vi "RTM - Add Packet.vi"() -> ()   [LabVIEW 2015, in "UDP-Custom-Device System Explorer.lvlib"]
uses:
  UDP-Custom-Device System Explorer.lvlib
  Shared/Constants.vi
  <vilib>/NI Veristand/Custom Device API/Get Item Property (String Array).vi
  <vilib>/NI Veristand/Custom Device API/Set Item Property (String Array).vi
  <vilib>/NI VeriStand/Custom Device API/Custom Device API.lvlib
  Shared/UDP-Custom-Device Shared.lvlib
  <vilib>/NI VeriStand/Custom Device Tools/Custom Device Utility Library/Custom Device Utility Library.lvlib
panel:
  in  "Cancel Button":bool
  in  "OK Button":bool
  in  "New Packet ID":string
  in  "New Packet Name":string
  in  "Tag":string
  in  "Node Ptr":u64 format="%.0x"
  out "error out":errorcluster
  in  "error in (no error)":errorcluster
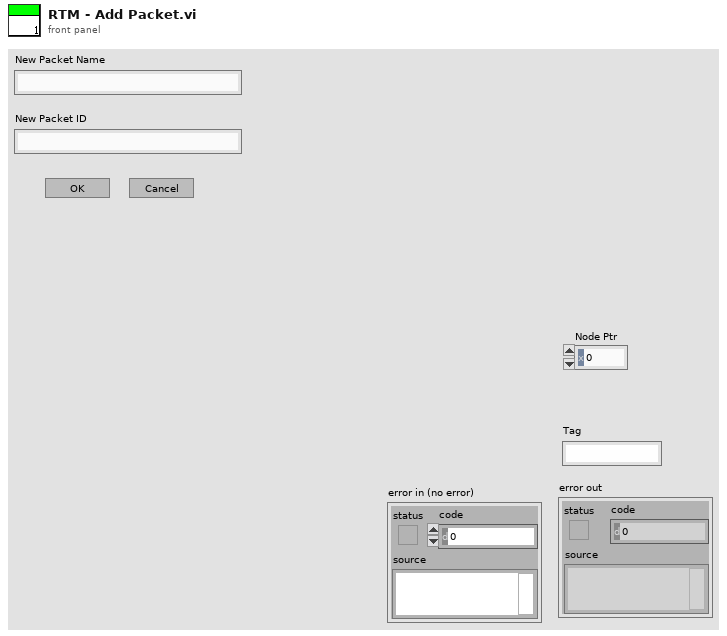
[diagram p1: front panel]
types:
  T1 = enum32{"Invalid", "Standard", "Closed", "Hidden", "Minimized", "Maximized"}
  T2 = typedef "Custom Device API.lvlib/Custom Device Item Ref.ctl" = u64
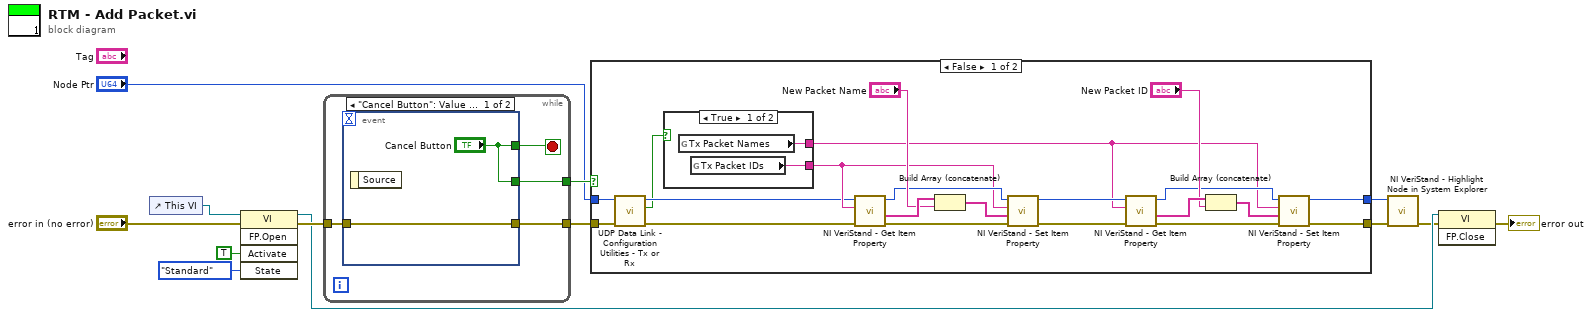
[diagram p0: block diagram]
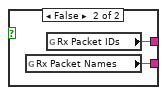
[diagram p2: hidden frame]
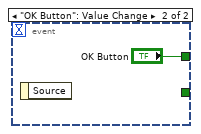
[diagram p4: hidden frame]
diagram:
  n1 = control-ref of="This VI"() -> (w13:refnum<vi>)
  n2 = invoke class="VI" method="FP.Open"(reference=w13, error in="error in (no error)", "Activate"=TRUE ("Activate?"), "State"=T1."Standard") -> (reference out=w4:refnum<vi>, error out=w9:errorcluster)  [unwired: 1 in, 3 out]
  n3 = while {
    tunnel: w9 -> [w16]
    tunnel: [w15] -> w7
    tunnel: [w14] -> w8
    stop <- w17 stop-if-true
    n4 = event shown="[0] \"Cancel Button\": Value Change" {
      selector: _ -> [_ _]
      dyn-events: _ -> [_ _]
      timeout: _ -> [_ _]
      tunnel: ["Cancel Button" "OK Button"] -> w17
      tunnel: w16 -> [w19 _]
      tunnel: [w19 _] -> w15
      tunnel: ["Cancel Button" _] -> w14
      event "Cancel Button": Value Change {
        n5 = event-data() -> ()  [unwired: 1 in, 1 out]
      }
      event "OK Button": Value Change {
        n6 = event-data() -> ()  [unwired: 1 in, 1 out]
      }
    }
  }
  n7 = case shown="False" w8 {
    tunnel: w7 -> [w25 w47]
    tunnel: [w31 w47] -> w3
    tunnel: "Node Ptr" -> [w26 w46]
    tunnel: [w21 w46] -> w1
    frame False {
      n8 = call "UDP Data Link - Configuration Utilities - Tx or Rx.vi"("error in (no error)"=w25, "Item Ref in"=w26) -> ("error out"=w24:errorcluster, "Tx?"=w22:bool, "Item Ref out"=w23:T2)  [unwired: 7 in]
      n9 = case shown="True" w22 {
        tunnel: [w43 w45] -> w28
        tunnel: [w42 w44] -> w27
        frame True {
          n10 = global read "Constants.vi" "Tx Packet Names"() -> (w42:string)
          n11 = global read "Constants.vi" "Tx Packet IDs"() -> (w43:string)
        }
        frame False {
          n12 = global read "Constants.vi" "Rx Packet Names"() -> (w45:string)
          n13 = global read "Constants.vi" "Rx Packet IDs"() -> (w44:string)
        }
      }
      n14 = call-poly <vilib>:"NI VeriStand - Get Item Property.vi"("error in (no error)"=w24, "Property Name"=w28, "Item Ref in"=w23) -> ("error out"=w41:errorcluster, "Value"=w40:string[], "Item Ref out"=w30:T2)  [unwired: 5 in, 1 out]
      n15 = Build Array (concatenate)(w40, "New Packet Name") -> (w39:string[])
      n16 = call-poly <vilib>:"NI VeriStand - Set Item Property.vi"("error in (no error)"=w41, "Value"=w39, "Property Name"=w28, "Item Ref in"=w30) -> ("error out"=w34:errorcluster, "Item Ref out"=w33:T2)  [unwired: 5 in, 1 out]
      n17 = call-poly <vilib>:"NI VeriStand - Get Item Property.vi"("error in (no error)"=w34, "Property Name"=w27, "Item Ref in"=w33) -> ("error out"=w35:errorcluster, "Value"=w36:string[], "Item Ref out"=w29:T2)  [unwired: 5 in, 1 out]
      n18 = Build Array (concatenate)(w36, "New Packet ID") -> (w37:string[])
      n19 = call-poly <vilib>:"NI VeriStand - Set Item Property.vi"("error in (no error)"=w35, "Value"=w37, "Property Name"=w27, "Item Ref in"=w29) -> ("error out"=w31:errorcluster, "Item Ref out"=w21:T2)  [unwired: 5 in, 1 out]
    }
    frame True {
    }
  }
  n20 = call <vilib>:"NI VeriStand - Highlight Node in System Explorer.vi"("error in (no error)"=w3, "Item Ref in"=w1) -> ("error out"=w2:errorcluster)  [unwired: 8 in, 1 out]
  n21 = invoke class="VI" method="FP.Close"(reference=w4, error in=w2) -> (error out=→"error out":errorcluster)  [unwired: 1 in, 2 out]
